vi "Bus Cycle--constant.vi"() -> (0 "Bus Cycle (microsecond)":u32)   [LabVIEW 2024, in "EtherCAT Model.lvlib"]
uses:
  EtherCAT Model.lvlib
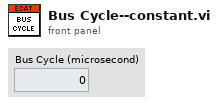
[diagram p1: front panel]
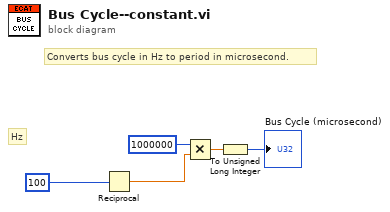
[diagram p0: block diagram]
diagram:
  # "Converts bus cycle in Hz to period in microsecond."
  # "Hz"
  n1 = Reciprocal(x=100) -> (1/x=w3:dbl)
  n2 = Multiply(x=1000000, y=w3) -> (x*y=w2:dbl)
  n3 = To Unsigned Long Integer(number=w2) -> (unsigned 32bit integer=→"Bus Cycle (microsecond)":u32)
